vi "CleanUpTemplateMethods_ReplaceErrorCluster.vi"(9 "SourceErrorCluster":refnum<vi>, 10 "NewErrorClusterCtlFile":path, 11 "TargetErrorClusterToReplace":refnum<vi>) -> (3 "newErrorCluster":refnum<vi>)   [LabVIEW 2020]
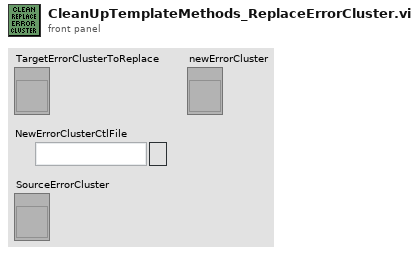
[diagram p1: front panel]
types:
  T1 = typedef "LVBoundsTypeDef.ctl" = cluster{"Width":u32, "Height":u32}
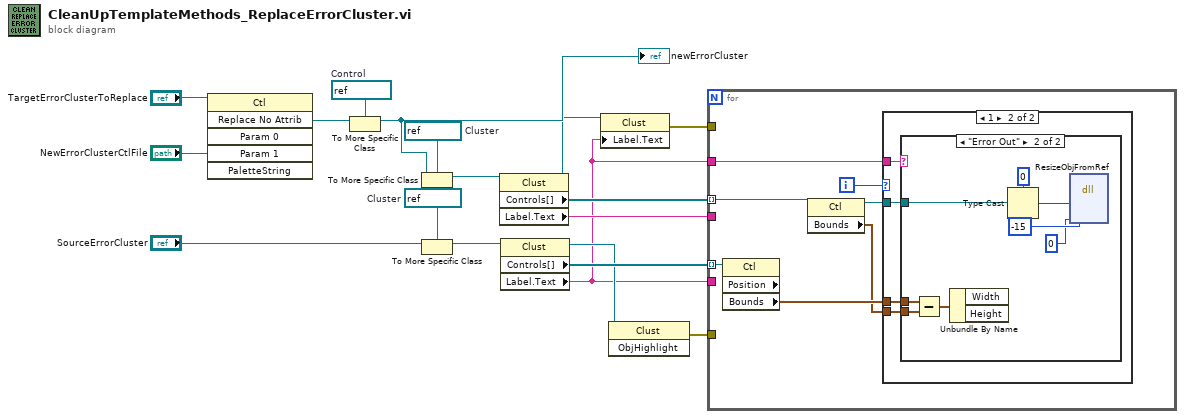
[diagram p0: block diagram]
diagram:
  w12 = refnum<vi> refnum  # Cluster
  w13 = refnum<vi> refnum  # Cluster
  w18 = refnum<vi> refnum  # Control
  n1 = invoke class="Ctl" method="Replace No Attrib"(reference="TargetErrorClusterToReplace", "Param 1"="NewErrorClusterCtlFile") -> ("RepNoAttrib"=w17:refnum<vi>)  [unwired: 4 in, 5 out]
  n2 = To More Specific Class(target class=w18, reference=w17) -> (specific class reference=w14:refnum<vi>)  [unwired: 1 in, 1 out]
  "newErrorCluster" <- w14
  n3 = To More Specific Class(target class=w13, reference=w14) -> (specific class reference=w10:refnum<vi>)  [unwired: 1 in, 1 out]
  n4 = To More Specific Class(target class=w12, reference="SourceErrorCluster") -> (specific class reference=w9:refnum<vi>)  [unwired: 1 in, 1 out]
  n5 = property class="Clust"(reference=w10) -> (reference out=w5:refnum<vi>, "Controls[]"=w8:refnum<vi>[], "Label.Text"=w6:string)  [unwired: 1 in, 1 out]
  n6 = property class="Clust"(reference=w9) -> (reference out=w3:refnum<vi>, "Controls[]"=w7:refnum<vi>[], "Label.Text"=w1:string)  [unwired: 1 in, 1 out]
  n7 = property class="Clust"(reference=w5, "Label.Text"=w1) -> (error out=w4:errorcluster)  [unwired: 1 in, 1 out]
  n8 = invoke class="Clust" method="ObjHighlight"(reference=w3) -> (error out=w2:errorcluster)  [unwired: 2 in, 2 out]
  n9 = for {
    tunnel: w8 -> [w25] mode=indexing
    tunnel: w7 -> [w24] mode=indexing
    tunnel: w1 -> [_]
    tunnel: w6 -> [_]
    tunnel: w4 -> [_]
    tunnel: w2 -> [_]
    tunnel: w1 -> [w19]
    i -> [w23]
    n10 = property class="Ctl" props=["Position", "Bounds"](reference=w24) -> ("Bounds"=w21:T1)  [unwired: 1 in, 3 out]
    n11 = property class="Ctl"(reference=w25) -> (reference out=w22:refnum<vi>, "Bounds"=w20:T1)  [unwired: 1 in, 1 out]
    n12 = case shown="1" w23 {
      tunnel: w22 -> [_ w27]
      tunnel: w21 -> [_ w29]
      tunnel: w20 -> [_ w28]
      tunnel: w19 -> [_ w26]
      frame 0, Default {
      }
      frame 1 {
        n13 = case shown="\"Error Out\"" w26 {
          tunnel: w29 -> [_ w35]
          tunnel: w28 -> [_ w34]
          tunnel: w27 -> [_ w31]
          frame Default {
          }
          frame "Error Out" {
            n14 = Subtract(x=w35, y=w34) -> (x-y=w30:T1)
            n15 = Unbundle By Name(w30) -> ()  [unwired: 2 out]
            n16 = Type Cast(type=0, x=w31) -> (*(type *) &x=w36:i32)
            n17 = dll-call lib="LabVIEW" fn="ResizeObjFromRef"("ref"=w36, "deltaHoriz"=-15, "deltaVert"=0) -> ()  [unwired: 6 in, 3 out]
          }
        }
      }
    }
  }
